vi "Find_total_cash.vi"(0 "Cash":T1) -> (4 "Total_Cash":i32)   [LabVIEW 2023, in "Vending_machine.lvlib"]
doc: "Used fine the cash amount from the bills present"
uses:
  Vending_machine.lvlib
  Controls/Cash.ctl
  Controls/Denominations.ctl
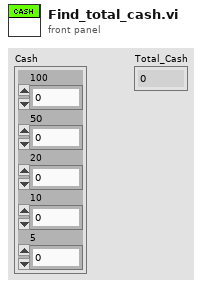
[diagram p1: front panel]
types:
  T1 = typedef "Vending_machine.lvlib/Cash.ctl" = cluster{"100":i32, "50":i32, "20":i32, "10":i32, "5":i32}
  T2 = typedef "Vending_machine.lvlib/Denominations.ctl" = string[]
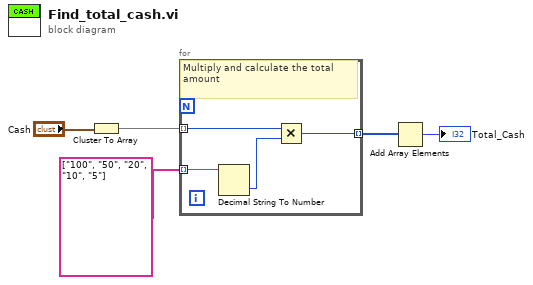
[diagram p0: block diagram]
diagram:
  n1 = Cluster To Array(cluster="Cash") -> (array=w4:i32[])
  n2 = for {
    tunnel: w4 -> [w8] mode=indexing
    tunnel: T2 ["100", "50", "20", "10", "5"] ("Array") -> [w9] mode=indexing
    tunnel: [w6] -> w2 mode=indexing
    # "Multiply and calculate the total amount"
    n3 = Decimal String To Number(string=w9) -> (number=w7:i32)  [unwired: 2 in, 1 out]
    n4 = Multiply(x=w8, y=w7) -> (x*y=w6:i32)
  }
  n5 = Add Array Elements(numeric array=w2) -> (sum=→"Total_Cash":i32)
